vi "run_date_fgv .vi"(2 "error in (no error)":errorcluster, 3 "mode":enum16{"read", "write"}(ring), 4 "DATE in":cluster{"电源电流A":dbl, bool, "VI":dbl, bool}) -> (0 "error out":errorcluster, 1 "DATE OUT":cluster{"电源电流A":dbl, bool, "VI":dbl, bool})   [LabVIEW 2019]
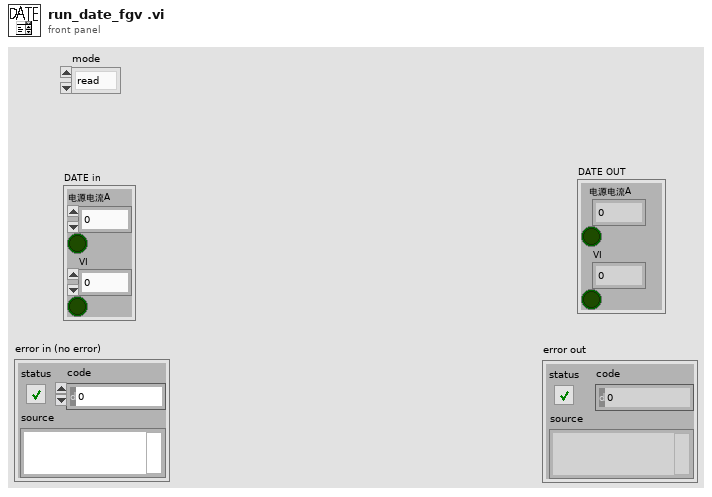
[diagram p1: front panel]
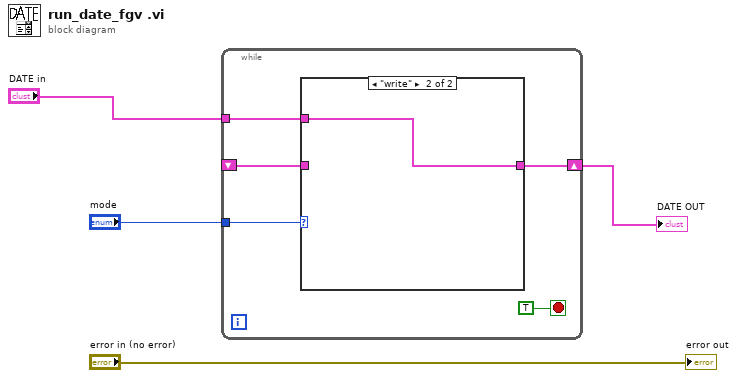
[diagram p0: block diagram]
diagram:
  n1 = while {
    tunnel: "mode" -> [w9]
    tunnel: "DATE in" -> [w8]
    shift-right: [w7] -> w1
    shift-left: _ -> [w6]
    stop <- TRUE stop-if-true
    n2 = case shown="\"write\"" w9 {
      tunnel: [w10 w11] -> w7
      tunnel: w8 -> [_ w11]
      tunnel: w6 -> [w10 _]
      frame "read", Default {
      }
      frame "write" {
      }
    }
  }
  "DATE OUT" <- w1
  "error out" <- "error in (no error)"
